vi "Write Direction.vi"(8 "error in (no error)":errorcluster, 10 "Direction":T1, 11 "AndrewF in":refnum<class "AndrewF.lvclass">) -> (0 "error out":errorcluster, 3 "AndrewF out":refnum<class "AndrewF.lvclass">)   [LabVIEW 2015, in "AndrewF.lvclass"]
uses:
  AndrewF.lvclass
  Type Defs/Direction Enum.ctl
  AndrewF.lvclass/AndrewF.ctl
  Type Defs/SB Type Defs.lvlib
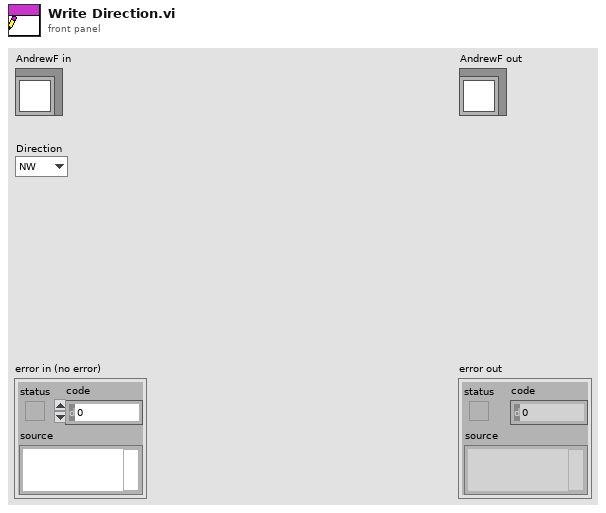
[diagram p1: front panel]
types:
  T1 = typedef "SB Type Defs.lvlib/Direction Enum.ctl" = enum16{"NW", "N", "NE", "E", "SE", "S", "SW", "W"}
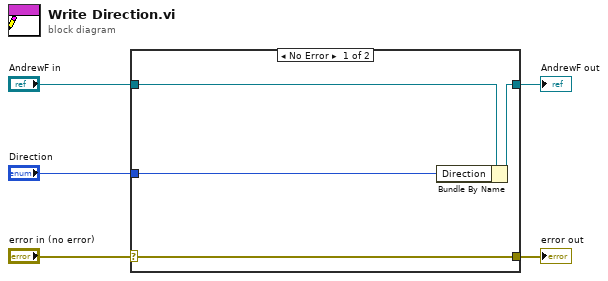
[diagram p0: block diagram]
diagram:
  n1 = case shown="No Error" "error in (no error)" {
    selector: "error in (no error)" -> [w9 w10]
    tunnel: [w9 w10] -> w4
    tunnel: [w7 w11] -> w2
    tunnel: "AndrewF in" -> [w8 w11]
    tunnel: "Direction" -> [w6 _]
    frame No Error {
      n2 = Bundle By Name(cluster=w8, "Direction"=w6) -> (w7:refnum<class "AndrewF.lvclass">)
    }
    frame Error {
    }
  }
  "error out" <- w4
  "AndrewF out" <- w2
